vi "target3.vi"() -> ()   [LabVIEW 2023]
panel:
  in  "size":i32=100
  out "evenNumbers":i32[](array[numeric])
  out "sum":i32
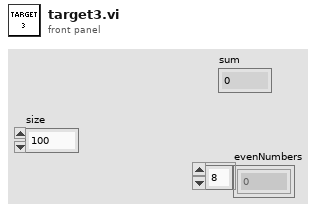
[diagram p1: front panel]
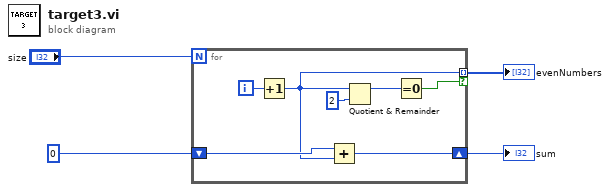
[diagram p0: block diagram]
diagram:
  n1 = for {
    N: "size" -> [_]
    shift-right: [w7] -> w2
    shift-left: 0 -> [w11]
    tunnel: [w5] -> w1 mode=indexing if=w6
    i -> [w10]
    n2 = Increment(x=w10) -> (x+1=w5:i32)
    n3 = Add(x=w11, y=w5) -> (x+y=w7:i32)
    n4 = Quotient & Remainder(x=w5, y=2) -> (x-y*floor(x/y)=w8:i32)  [unwired: 1 out]
    n5 = Equal To 0?(x=w8) -> (x = 0?=w6:bool)
  }
  "sum" <- w2
  "evenNumbers" <- w1
